vi "Pockels Cal-Call zero entry dialogue.vi"(11 "Measured Power":dbl caption="Enter Measured Power (mW)" min=0.0 max=10000.0 step=1.0 format="%#_6f") -> (3 "Next (ind)":bool)   [LabVIEW 2017]
uses:
  Globals/gl_Calibration globals.vi
types:
  T1 = typedef "Pockels cal process refs.ctl" = cluster{"This VI":refnum<vi>, "Abort (ind)":refnum<vi>, "Next (ind)":refnum<vi>, "Cancel":refnum<vi>, "Next":refnum<vi>, "Message":refnum<vi>, "Measured Power ctrl":refnum<vi>, "Measured Power ind":refnum<vi>, "Pockels cal progress bar":refnum<vi>, "Abort this objective":refnum<vi>}
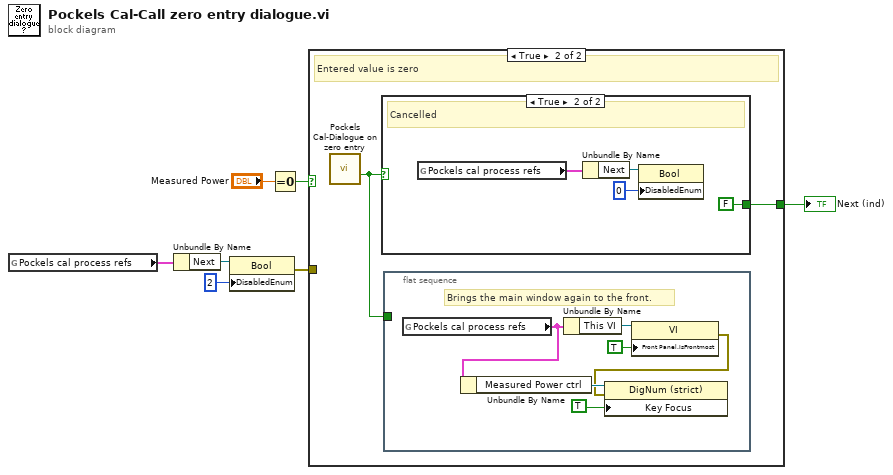
[diagram p0: block diagram]
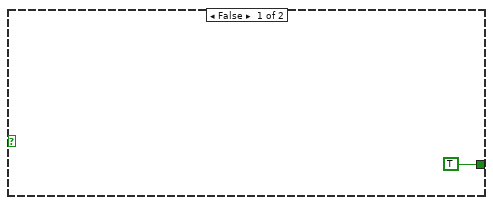
[diagram p2: hidden frame]
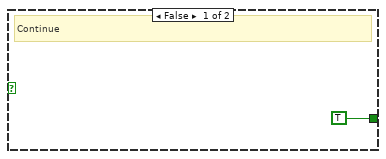
[diagram p3: hidden frame]
diagram:
  n1 = global read "gl_Calibration globals.vi" "Pockels cal process refs"() -> (w2:T1)
  n2 = Unbundle By Name(w2) -> ("Next"=w4:refnum<vi>)
  n3 = property class="Bool"(reference=w4, "DisabledEnum"=2) -> (error out=w1:errorcluster)  [unwired: 1 in, 1 out]
  n4 = Equal To 0?(x="Measured Power") -> (x = 0?=w5:bool)
  n5 = case shown="True" w5 {
    tunnel: [TRUE ("Next (ind)") w10] -> w7
    tunnel: w1 -> [_ _]
    frame False {
    }
    frame True {
      # "Entered value is zero"
      n6 = call "Pockels Cal-Dialogue on zero entry.vi"() -> ("Cancelled (Left button pressed)"=w9:bool)  [unwired: 10 in, 1 out]
      n7 = case shown="True" w9 {
        tunnel: [TRUE ("Next (ind)") FALSE ("Next (ind)")] -> w10
        frame False {
          # "Continue"
        }
        frame True {
          # "Cancelled"
          n8 = global read "gl_Calibration globals.vi" "Pockels cal process refs"() -> (w20:T1)
          n9 = Unbundle By Name(w20) -> ("Next"=w18:refnum<vi>)
          n10 = property class="Bool"(reference=w18, "DisabledEnum"=0) -> ()  [unwired: 1 in, 2 out]
        }
      }
      n11 = flat-sequence {
        tunnel: w9 -> [_]
        frame #0 {
          # "Brings the main window again to the front."
          n12 = global read "gl_Calibration globals.vi" "Pockels cal process refs"() -> (w11:T1)
          n13 = Unbundle By Name(w11) -> ("Measured Power ctrl"=w14:refnum<vi>)
          n14 = Unbundle By Name(w11) -> ("This VI"=w15:refnum<vi>)
          n15 = property on="Property Node" class="VI"(reference=w15, "Front Panel.IsFrontmost"=TRUE ("Front Panel Window:Is Frontmost")) -> (error out=w13:errorcluster)  [unwired: 1 in, 1 out]
          n16 = property on="Property Node" class="DigNum (strict)"(reference=w14, error in=w13, "Key Focus"=TRUE ("Front Panel Window:Is Frontmost")) -> ()  [unwired: 2 out]
        }
      }
    }
  }
  "Next (ind)" <- w7
